vi "draw.vi"(8 "error in (no error)":errorcluster, 11 "CompoundShape in":refnum<class "CompoundShape.lvclass">) -> (0 "error out":errorcluster, 3 "CompoundShape out":refnum<class "CompoundShape.lvclass">)   [LabVIEW 2018, in "CompoundShape.lvclass"]
uses:
  CompoundShape.lvclass
  Shape Class/Shape.lvclass
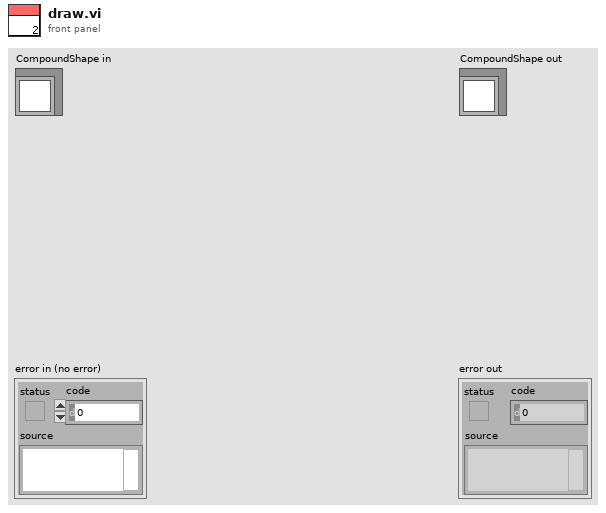
[diagram p1: front panel]
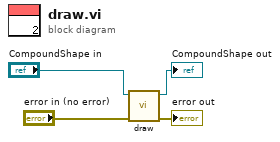
[diagram p0: block diagram]
diagram:
  n1 = call-parent "draw.vi"("error in (no error)"="error in (no error)", "Shape in"="CompoundShape in") -> ("error out"=→"error out":errorcluster, "Shape out"=→"CompoundShape out":refnum<class "CompoundShape.lvclass">)  [unwired: 8 in]
